vi "Tosca-Pause.vi"(0 "Pause ref":refnum<vi>, 11 "error in (no error)":errorcluster) -> (15 "error out":errorcluster)   [LabVIEW 2020]
uses:
  Trace VIs/Tosca-Trace-Event.ctl
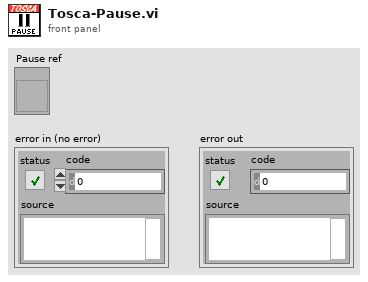
[diagram p1: front panel]
types:
  T1 = typedef "Tosca-Trace-Event.ctl" = enum16{"Unspecified", "Trial start", "Enqueue", "Result", "End parser", "Frame", "Queue available", "Timeout sent", "WritePos", "TTL"}
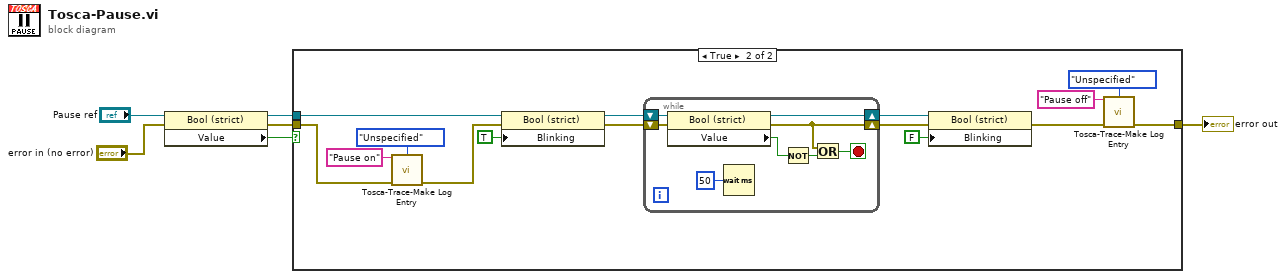
[diagram p0: block diagram]
diagram:
  n1 = property class="Bool (strict)"(reference="Pause ref", error in="error in (no error)") -> (reference out=w4:refnum<vi>, error out=w3:errorcluster, "Value"=w2:bool)
  n2 = case shown="True" w2 {
    tunnel: w4 -> [_ w22]
    tunnel: w3 -> [w7 w13]
    tunnel: [w7 w8] -> w1
    frame False {
    }
    frame True {
      n3 = call "Tosca-Trace-Make Log Entry.vi"("Message"="Pause on", "Event"=Tosca-Trace-Event."Unspecified", "error in (no error)"=w13) -> ("error out"=w12:errorcluster)  [unwired: 12 in]
      n4 = property class="Bool (strict)"(reference=w22, error in=w12, "Blinking"=TRUE) -> (reference out=w20:refnum<vi>, error out=w19:errorcluster)
      n5 = while {
        shift-right: [w24] -> w17
        shift-left: w19 -> [w26]
        shift-right: [w23] -> w16
        shift-left: w20 -> [w27]
        stop <- w25 stop-if-true
        n6 = property class="Bool (strict)"(reference=w27, error in=w26) -> (reference out=w23:refnum<vi>, error out=w24:errorcluster, "Value"=w30:bool)
        n7 = Wait (ms)(milliseconds to wait=u32 50) -> ()  [unwired: 1 out]
        n8 = Not(x=w30) -> (.not. x?=w29:bool)
        n9 = Or(x=w24, y=w29) -> (x .or. y?=w25:bool)
      }
      n10 = property class="Bool (strict)"(reference=w16, error in=w17, "Blinking"=FALSE) -> (error out=w9:errorcluster)  [unwired: 1 out]
      n11 = call "Tosca-Trace-Make Log Entry.vi"("Message"="Pause off", "Event"=Tosca-Trace-Event."Unspecified", "error in (no error)"=w9) -> ("error out"=w8:errorcluster)  [unwired: 12 in]
    }
  }
  "error out" <- w1
